vi "Start New Report.vi"(8 "error in (no error)":errorcluster, 10 "parameters":T1, 11 "Sequencer Module runtime in":refnum<class "Sequencer Module runtime.lvclass">) -> (0 "error out":errorcluster, 2 "Parameters allocation out":T1, 3 "Sequencer Module runtime out":refnum<class "Sequencer Module runtime.lvclass">)   [LabVIEW 2015, in "Sequencer Module runtime.lvclass"]
uses:
  Sequencer Module runtime.lvclass
  <vilib>/NI/Tag Bus/table/data table.ctl
  classes/Report Information/DUT Information.ctl
  classes/Report Information/Station Information.ctl
  classes/Report Information/Test Information.ctl
  Sequencer Module runtime.lvclass/Sequencer Module runtime.ctl
  classes/Result Processor/Execution/ResultProcessor.lvclass
  <vilib>/NI/Tag Bus/table/data table.lvlib
  classes/Report Information/Report Information.lvclass
panel:
  in  "Test Information":T2={"UUT Result"="Result"}
  in  "Station Info":T3={"Station ID"="Station43", "Station Serial Number"="sn123456n43"}
  in  "DUT Info":T4={"DUT Serial Number"="sn4455432", "DUT Info"="Batt45"}
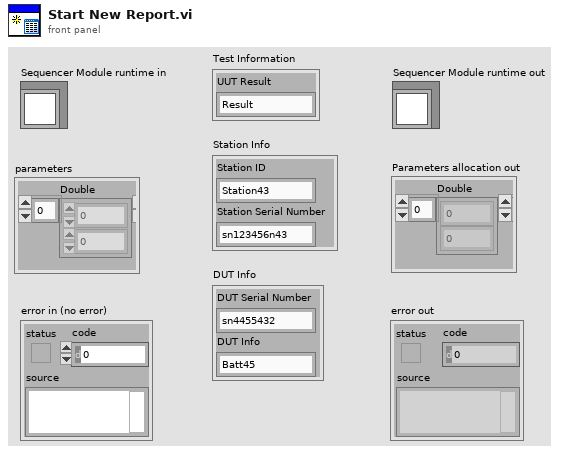
[diagram p1: front panel]
types:
  T1 = typedef "tag bus.lvlib/data table.lvlib/data table.ctl" = cluster{"Double":dbl[], "Single":sgl[], "I64":i64[], "I32":i32[], "I16":i16[], "I8":i8[], "U64":u64[], "U32":u32[], "U16":u16[], "U8":u8[], "Boolean":bool[], "String":string[], "Array of Double":cluster{"DBL Array":dbl[]}[], "Array of Single":cluster{"SGL Array":sgl[]}[], "Array of I64":cluster{"I64 Array":i64[]}[], "Array of I32":cluster{"I32 Array":i32[]}[], "Array of I16":cluster{"I16 Array":i16[]}[], "Array of I8":cluster{"I8 Array":i8[]}[], "Array of U64":cluster{"U64 Array":u64[]}[], "Array of U32":cluster{"U32 Array":u32[]}[], "Array of U16":cluster{"U16 Array":u16[]}[], "Array of U8":cluster{"U8 Array":u8[]}[], "Array of Boolean":cluster{"Boolean Array":bool[]}[], "Array of String":cluster{"String Array":string[]}[]}
  T2 = typedef "Report Information.lvclass/Test Information.ctl" = cluster{"UUT Result":string}
  T3 = typedef "Report Information.lvclass/Station Information.ctl" = cluster{"Station ID":string, "Station Serial Number":string}
  T4 = typedef "Report Information.lvclass/DUT Information.ctl" = cluster{"DUT Serial Number":string, "DUT Info":string}
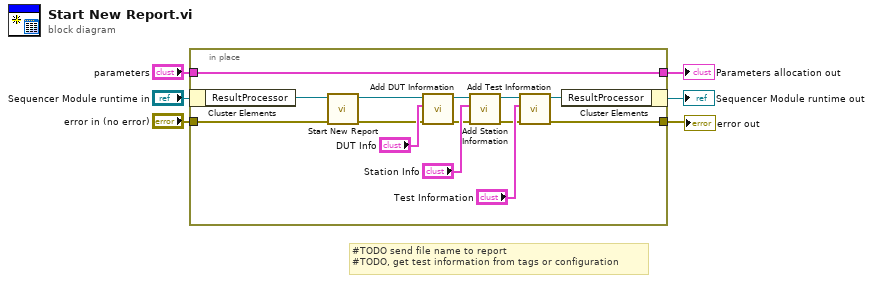
[diagram p0: block diagram]
diagram:
  # "#TODO send file name to report\n#TODO, get test information from tags or configuration"
  n1 = in-place {
    in-place-border: [w13] -> w4
    in-place-border: "parameters" -> [w13]
    in-place-border: [w8] -> w2
    in-place-border: "error in (no error)" -> [w7]
    n2 = in-place-cluster #1("Sequencer Module runtime in") -> ("ResultProcessor"=w14:refnum<class "ResultProcessor.lvclass">)
    n3 = call "Start New Report.vi"("error in (no error)"=w7, "ResultProcessor in"=w14) -> ("error out"=w11:errorcluster, "ResultProcessor out"=w19:refnum<class "ResultProcessor.lvclass">)  [unwired: 8 in]
    n4 = call "Add DUT Information.vi"("error in (no error)"=w11, "DUT Info"="DUT Info", "ResultProcessor in"=w19) -> ("error out"=w10:errorcluster, "ResultProcessor out"=w17:refnum<class "ResultProcessor.lvclass">)  [unwired: 7 in]
    n5 = call "Add Station Information.vi"("error in (no error)"=w10, "Station Info"="Station Info", "ResultProcessor in"=w17) -> ("error out"=w9:errorcluster, "ResultProcessor out"=w15:refnum<class "ResultProcessor.lvclass">)  [unwired: 7 in]
    n6 = call "Add Test Information.vi"("error in (no error)"=w9, "Test Information"="Test Information", "ResultProcessor in"=w15) -> ("error out"=w8:errorcluster, "ResultProcessor out"=w12:refnum<class "ResultProcessor.lvclass">)  [unwired: 7 in]
    n7 = in-place-cluster #1("ResultProcessor"=w12) -> (→"Sequencer Module runtime out":refnum<class "Sequencer Module runtime.lvclass">)
  }
  "Parameters allocation out" <- w4
  "error out" <- w2
